vi "Scan Setup.vi"(8 "error in (no error)":errorcluster, 11 "Instrument in":refnum<class "Instrument.lvclass">) -> (0 "error out":errorcluster, 1 "User Cancelled?":bool, 3 "Instrument out":refnum<class "Instrument.lvclass">)   [LabVIEW 2009, in "Instrument.lvclass"]
doc: "(Dynamic) Send commands to configure the instrument according to the class member fields."
uses:
  Instrument.lvclass
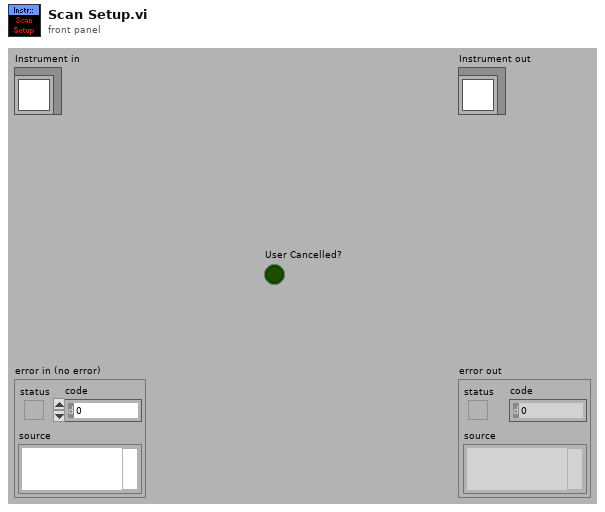
[diagram p1: front panel]
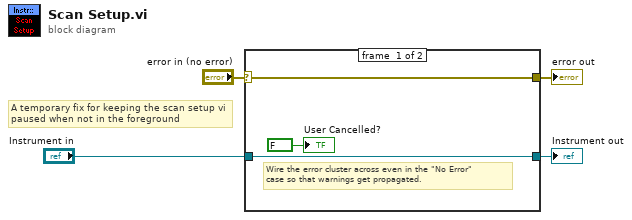
[diagram p0: block diagram]
diagram:
  # "A temporary fix for keeping the scan setup vi \npaused when not in the foreground"
  n1 = case shown="No Error" "error in (no error)" {
    selector: "error in (no error)" -> [w5 w9]
    tunnel: [w5 w9] -> w3
    tunnel: [w6 w8] -> w1
    tunnel: "Instrument in" -> [w6 w8]
    frame #0 {
      # "Wire the error cluster across even in the \"No Error\"\ncase so that warnings get propagated."
      "User Cancelled?" <- FALSE ("User Cancelled?")
    }
    frame #1 {
    }
  }
  "error out" <- w3
  "Instrument out" <- w1
